vi "生成文件.vi"(8 "错误输入（无错误）":errorcluster, 10 "通道个数":i32, 11 "数据":string[][](array[string])) -> (0 "error out":errorcluster)   [LabVIEW 2011]
uses:
  <vilib>/Utility/NIReport.llb/NI_report.lvclass
  <vilib>/addons/_office/excel.llb/Excel Easy Table (str).vi
  <vilib>/addons/_office/NI_ReportGenerationToolkit.lvlib
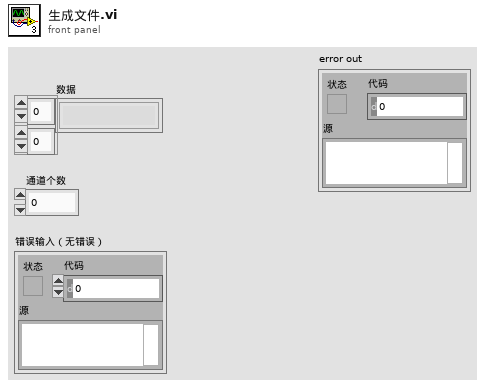
[diagram p1: front panel]
types:
  T1 = enum16{"maximized", "minimized", "normal", "no change"}
  T2 = enum16{"Standard Report", "HTML", "Word", "Excel"}
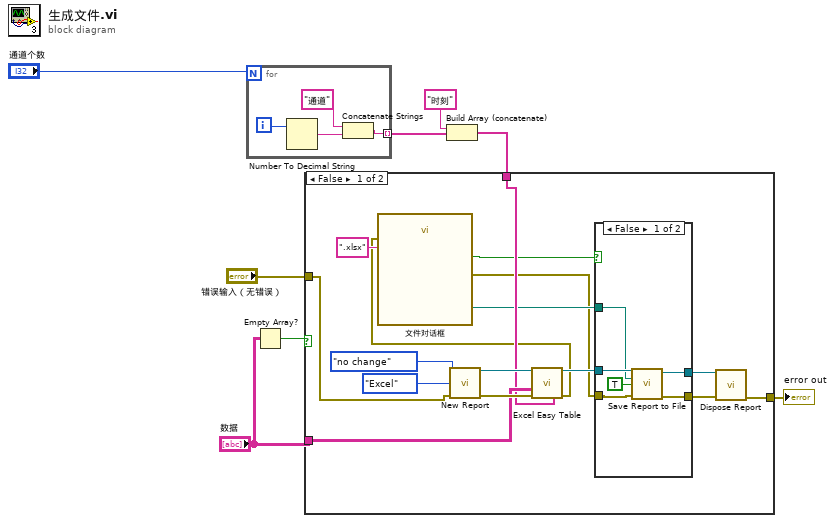
[diagram p0: block diagram]
diagram:
  n1 = for {
    N: "通道个数" -> [_]
    tunnel: [w9] -> w5 mode=indexing
    i -> [w12]
    n2 = Number To Decimal String(number=w12) -> (decimal integer string=w11:string)  [unwired: 1 in]
    n3 = Concatenate Strings("通道" ("字符串"), w11) -> (w9:string)
  }
  n4 = Empty Array?(array="数据") -> (empty?=w8:bool)
  n5 = Build Array (concatenate)("时刻", w5) -> (w6:string[])
  n6 = case shown="False" w8 {
    tunnel: "错误输入（无错误）" -> [w18 w37]
    tunnel: w6 -> [w20 _]
    tunnel: "数据" -> [w21 _]
    tunnel: [w13 w37] -> w1
    frame False {
      n7 = call <vilib>:"New Report.vi"("window state (normal)"=T1."no change", "report type"=T2."Excel", "error in (no error)"=w18) -> ("report out"=w24:refnum<class "NI_report.lvclass">, "error out"=w23:errorcluster)  [unwired: 11 in]
      n8 = call-poly <vilib>:"Excel Easy Table.vi"("report in"=w24, "text data"=w21, "error in (no error)"=w23, "column headers"=w20) -> ("report out"=w22:refnum<class "NI_report.lvclass">, "error out"=w15:errorcluster)  [unwired: 7 in, 3 out]
      n9 = call "文件对话框"("error in"=w15, "pattern (all files)"=".xlsx") -> ("selected path"=w17:path, "cancelled"=w16:bool, "error out"=w14:errorcluster)  [unwired: 10 in, 1 out]
      n10 = case shown="False" w16 {
        tunnel: [w34 w35] -> w27
        tunnel: [w33 w36] -> w26
        tunnel: w22 -> [w31 w36]
        tunnel: w14 -> [w30 w35]
        tunnel: w17 -> [w29 _]
        frame False {
          n11 = call-dynamic "Save Report to File.vi"("report in"=w31, "report file path"=w29, "prompt to replace? (F)"=TRUE, "error in (no error)"=w30) -> ("report out"=w33:refnum<class "NI_report.lvclass">, "error out"=w34:errorcluster)  [unwired: 10 in]
        }
        frame True {
        }
      }
      n12 = call-dynamic "Dispose Report.vi"("report in"=w26, "error in (no error)"=w27) -> ("error out"=w13:errorcluster)  [unwired: 13 in]
    }
    frame True {
    }
  }
  "error out" <- w1
